vi "readNotifierStatus.vi"(8 "error in (no error)":errorcluster, 9 "notifierStatusOld":bool, 10 "serverSelection":enum16{"cmd", "tel"}(ring), 11 "TcpServer in":refnum<class "TcpServer.lvclass">) -> (0 "error out (no error)":errorcluster, 1 "notifierStatusNew":bool, 3 "TcpServer out":refnum<class "TcpServer.lvclass">)   [LabVIEW 2018, in "TcpServer.lvclass"]
doc: "Read the notifier sent from tcpServerStateMachine.vi.\n\nNotes: \n1. Put this VI in Prealocated reentrant clone execution.\n2. This vi is public for test purspose only. Please don´t use this vi."
uses:
  TcpServer.lvclass
  TcpServer.lvclass/TcpServer.ctl
  TcpServerCmd/TcpServerCmd.lvclass
  home/pcortes/github/ts_labview_tcp_json/src/TcpServerBase/TcpServerBase.lvclass
  TcpServerTel/TcpServerTel.lvclass
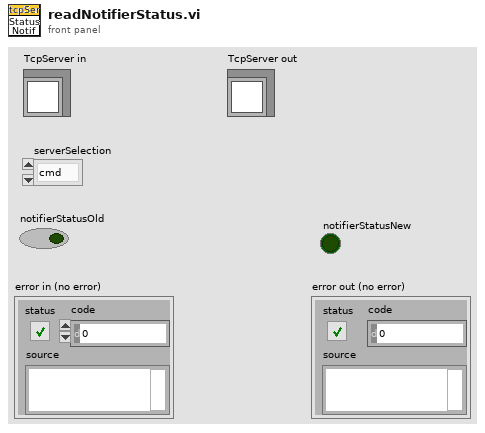
[diagram p1: front panel]
types:
  T1 = cluster{"connectionStatus":bool, "errorSource":string}
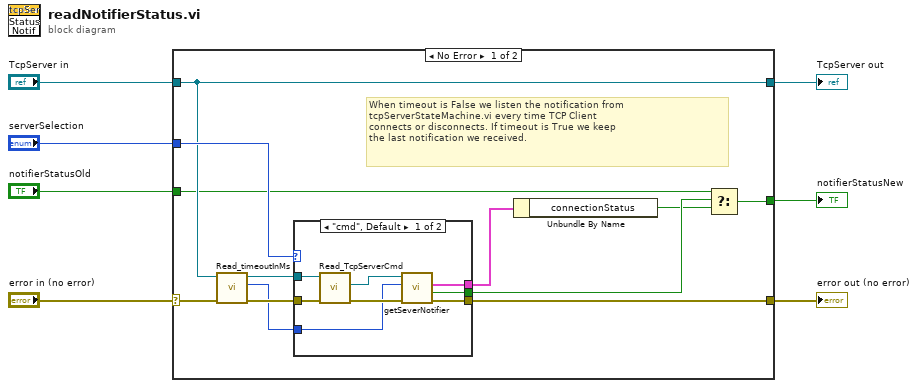
[diagram p0: block diagram]
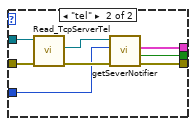
[diagram p2: hidden frame]
diagram:
  n1 = case shown="No Error" "error in (no error)" {
    selector: "error in (no error)" -> [w18 w37]
    tunnel: [w8 w38] -> w7
    tunnel: "notifierStatusOld" -> [w9 w38]
    tunnel: [w12 w37] -> w4
    tunnel: [w14 w36] -> w2
    tunnel: "TcpServer in" -> [w14 w36]
    tunnel: "serverSelection" -> [w19 _]
    frame No Error {
      # "When timeout is False we listen the notification from\ntcpServerStateMachine.vi every time TCP Client\nconnects or disconnects. If timeout is True we keep\nthe last notification we received."
      n2 = call "Read_timeoutInMs.vi"("error in (no error)"=w18, "TcpServer in"=w14) -> ("error out"=w17:errorcluster, "timeoutInMs"=w15:i32, "TcpServer out"=w16:refnum<class "TcpServer.lvclass">)  [unwired: 7 in]
      n3 = case shown="\"cmd\", Default" w19 {
        tunnel: w17 -> [w26 w35]
        tunnel: w16 -> [w27 w34]
        tunnel: w15 -> [w23 w29]
        tunnel: [w22 w30] -> w13
        tunnel: [w21 w31] -> w11
        tunnel: [w20 w32] -> w12
        frame "cmd", Default {
          n4 = call "Read_TcpServerCmd.vi"("error in (no error)"=w26, "TcpServer in"=w27) -> ("error out"=w25:errorcluster, "TcpServerCmd.lvclass"=w24:refnum<class "TcpServerCmd.lvclass">)  [unwired: 7 in, 1 out]
          n5 = call "getSeverNotifier.vi"("error in (no error)"=w25, "notifier timeout"=w23, "TcpServerBase in"=w24) -> ("error out"=w20:errorcluster, "timeout?"=w21:bool, "connStatusCluster"=w22:T1)  [unwired: 5 in, 1 out]
        }
        frame "tel" {
          n6 = call "Read_TcpServerTel.vi"("error in (no error)"=w35, "TcpServer in"=w34) -> ("error out"=w33:errorcluster, "TcpServerTel.lvclass"=w28:refnum<class "TcpServerTel.lvclass">)  [unwired: 7 in, 1 out]
          n7 = call "getSeverNotifier.vi"("error in (no error)"=w33, "Timeout Notifier"=w29, "TcpServerBase in"=w28) -> ("error out"=w32:errorcluster, "connStatus"=w31:bool, "connStatusCluster"=w30:T1)  [unwired: 5 in, 1 out]
        }
      }
      n8 = Unbundle By Name(w13) -> ("connectionStatus"=w10:bool)
      n9 = Select(t=w9, s=w11, f=w10) -> (s? t:f=w8:bool)
    }
    frame Error {
    }
  }
  "notifierStatusNew" <- w7
  "error out (no error)" <- w4
  "TcpServer out" <- w2
